vi "event_setup_toggle.vi"(7 "NewVal":bool, 8 "error in":errorcluster, 9 "reference cluster in":T1, 11 "Boolean in":refnum<vi>) -> (0 "error out":errorcluster)   [LabVIEW 2016]
uses:
  Type Definitions/reference_cluster.ctl
  Type Definitions/vars_settings.ctl
  Type Definitions/stim_type.ctl
  Type Definitions/backlight_type.ctl
  Type Definitions/vars_runtime.ctl
  Type Definitions/data.ctl
  Type Definitions/notifier_elements_GUI.ctl
  Type Definitions/notifier_elements_DAQ.ctl
  Type Definitions/notifier_elements_write.ctl
  Type Definitions/control_references.ctl
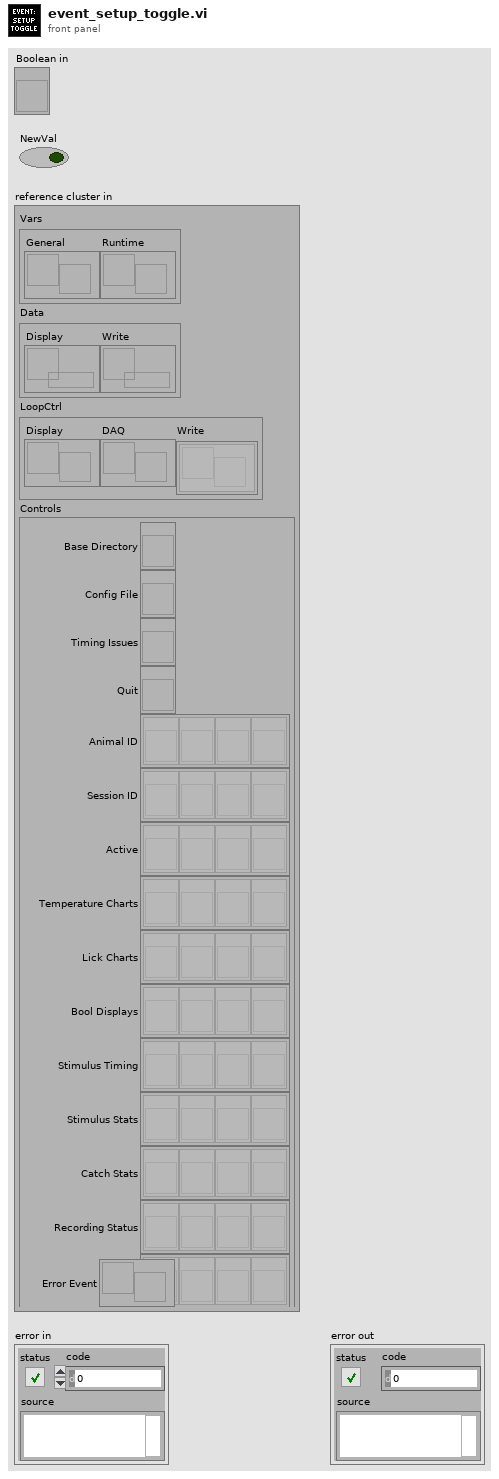
[diagram p1: front panel]
types:
  T1 = typedef "reference_cluster.ctl" = cluster{"Vars":cluster{"General":refnum<notifier>, "Runtime":refnum<notifier>}, "Data":cluster{"Display":refnum<queue>, "Write":refnum<queue>}, "LoopCtrl":cluster{"Display":refnum<notifier>, "DAQ":refnum<notifier>, "Write":refnum<notifier>[]}, "Controls":T2, "Error Event":refnum<user-event>}
  T2 = typedef "control_references.ctl" = cluster{"Base Directory":refnum<vi>, "Config File":refnum<vi>, "Timing Issues":refnum<vi>, "Quit":refnum<vi>, "Animal ID":refnum<vi>[], "Session ID":refnum<vi>[], "Active":refnum<vi>[], "Temperature Charts":refnum<vi>[], "Lick Charts":refnum<vi>[], "Bool Displays":refnum<vi>[], "Stimulus Timing":refnum<vi>[], "Stimulus Stats":refnum<vi>[], "Catch Stats":refnum<vi>[], "Recording Status":refnum<vi>[], "Pairing":refnum<vi>[]}
  T3 = typedef "vars_settings.ctl" = cluster{"base directory":path, "data directory":path, "active":bool, "running":bool, "pairing":bool, "clean tubes":bool, "animal ID":u16, "session ID":u16, "base temp":dbl, "d wait min":u16, "d wait max":u16, "d timeout":u16, "d timeout catch":u16, "d penalty":u16, "d reward":u16, "n reward":u16, "idx stim":u16, "timeout win":u16, "lick win":i32[], "stim type":T4[], "stim dur":u16[], "stim amp":dbl[], "stim freq":u16[], "stim ramp":u16[], "stim catch":u8[], "pairing delay":i16[], "square dur":u16[], "square delay":i16[], "square freq":u8[], "square dc":u8[], "stim shape":dbl[][], "square shape":bool[][], "backlight type":T5, "backlight freq":u16, "dStimOne dur":u16[], "dStimOne delay":i16[], "dStimTwo dur":u16[], "dStimTwo delay":i16[]}
  T4 = typedef "stim_type.ctl" = enum16{"pulse", "vibration", "square", "sine"}
  T5 = typedef "backlight_type.ctl" = enum16{"none", "random", "regular"}
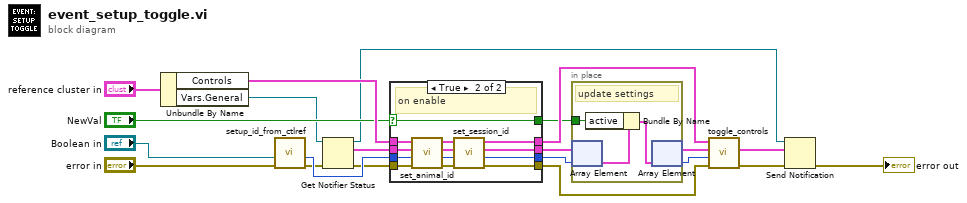
[diagram p0: block diagram]
diagram:
  n1 = Unbundle By Name("reference cluster in") -> ("Controls"=w12:T2, "Vars.General"=w4:refnum<notifier>)
  n2 = call "setup_id_from_ctlref.vi"("error in"="error in", "Ctl Refnum"="Boolean in") -> ("error out"=w7:errorcluster, "setup ID"=w11:u16)  [unwired: 6 in]
  n3 = Get Notifier Status(notifier=w4, error in (no error)=w7) -> (notifier out=w1:refnum<notifier>, current notification=w8:T3[], error out=w9:errorcluster)  [unwired: 2 out]
  n4 = case shown="True" "NewVal" {
    selector: "NewVal" -> [w23 w31]
    tunnel: [w25 w35] -> w16
    tunnel: w9 -> [w25 w34]
    tunnel: w12 -> [w22 w33]
    tunnel: w8 -> [w26 w27]
    tunnel: [w26 w32] -> w15
    tunnel: w11 -> [w24 w29]
    tunnel: [w23 w31] -> w13
    tunnel: [w24 w30] -> w14
    tunnel: [w22 w28] -> w21
    frame False {
      # "on disable"
    }
    frame True {
      # "on enable"
      n5 = call "set_animal_id.vi"("error in"=w34, "setup ID"=w29, "settings array in"=w27, "control cluster in"=w33) -> ("error out"=w39:errorcluster, "setup ID"=w37:u16, "settings array out"=w38:T3[], "control cluster out"=w36:T2)  [unwired: 2 in]
      n6 = call "set_session_id.vi"("control cluster in"=w36, "settings in"=w38, "setup ID"=w37, "error in"=w39) -> ("control cluster out"=w28:T2, "settings out"=w32:T3[], "Setup ID"=w30:i32, "error out"=w35:errorcluster)  [unwired: 3 in]
    }
  }
  n7 = in-place {
    in-place-border: w13 -> [w41]
    # "update settings"
    n8 = in-place-array #1(w15, w14) -> (w42:T3)
    n9 = Bundle By Name(cluster=w42, "active"=w41) -> (w40:T3)
    n10 = in-place-array #1(w40) -> (w20:T3[], w19:i32)
  }
  n11 = call "toggle_controls.vi"("error in"=w16, "setup ID"=w19, "vars general in"=w20, "control cluster in"=w21) -> ("error out"=w17:errorcluster, "vars general out"=w18:T3[])  [unwired: 4 in, 2 out]
  n12 = Send Notification(notification=w18, notifier=w1, error in (no error)=w17) -> (error out=→"error out":errorcluster)  [unwired: 1 out]
